vi "[Test] Put file.vi"() -> ()   [LabVIEW 2016, in "Tests.lvlib"]
uses:
  Tests.lvlib
  Protocol.ctl
  classes/File Transfer Behavior/File Transfer Behavior.lvclass
panel:
  in  "Password":string
  in  "Username":string
  in  "Protocol":T1
  in  "Address":string
  in  "Local path":path
  in  "Remote path":string
  out "error out":errorcluster
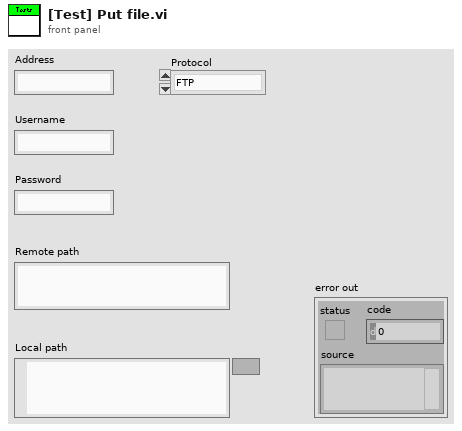
[diagram p1: front panel]
types:
  T1 = typedef "Tests.lvlib/Protocol.ctl" = enum16{"FTP", "WebDAV"}
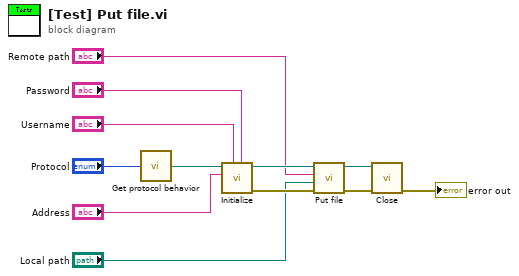
[diagram p0: block diagram]
diagram:
  n1 = call "Get protocol behavior.vi"("Protocol"="Protocol") -> ("RT Management.lvlib:FTP.lvclass"=w12:refnum<class "File Transfer Behavior.lvclass">)
  n2 = call-dynamic "Initialize.vi"("Password"="Password", "Username"="Username", "Address"="Address", "File Transfer Behavior in"=w12) -> ("error out"=w11:errorcluster, "File Transfer Behavior out"=w10:refnum<class "File Transfer Behavior.lvclass">)  [unwired: 6 in]
  n3 = call-dynamic "Put file.vi"("error in (no error)"=w11, "Local path"="Local path", "Remote path"="Remote path", "File Transfer Behavior in"=w10) -> ("error out"=w9:errorcluster, "File Transfer Behavior out"=w8:refnum<class "File Transfer Behavior.lvclass">)  [unwired: 6 in]
  n4 = call-dynamic "Close.vi"("error in (no error)"=w9, "File Transfer Behavior in"=w8) -> ("error out"=→"error out":errorcluster)  [unwired: 9 in]
